vi "terminate.vi"(0 "reference in":refnum<class "Master Controller.lvclass">, 5 "error in (no error)":errorcluster) -> (14 "reference out":refnum<class "Master Controller.lvclass">, 19 "error out":errorcluster)   [LabVIEW 2016, in "Master Controller.lvclass"]
uses:
  Master Controller.lvclass
  File Controller_llb/File Controller.lvclass
  Devices Controller_llb/Devices Controller.lvclass
  Items Controller_llb/Items Controller.lvclass
  PartsTracking Controller_class/PartsTracking Controller.lvclass
  GUI/GUI Controller_llb/GUI Controller.lvclass
  Notification Controller_class/Notification Controller.lvclass
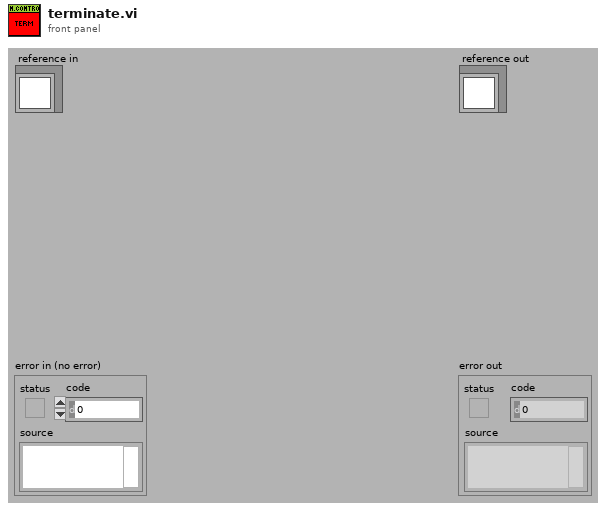
[diagram p1: front panel]
types:
  T1 = typedef "Master Controller.lvclass/ObjectAttributesRef.ctl" = refnum<data-value>
  T2 = typedef "Master Controller.lvclass/ObjectAttributes.ctl" = cluster{"MyAttribute":dbl, "Devices Controller_ref":refnum<class "Devices Controller.lvclass">, "File Controller_ref":refnum<class "File Controller.lvclass">, "Items Controller_ref":refnum<class "Items Controller.lvclass">, "GUI Controller_ref":refnum<class "GUI Controller.lvclass">, "NotificationController_ref":refnum<class "Notification Controller.lvclass">, "PartsTracking Controller_ref":refnum<class "PartsTracking Controller.lvclass">}
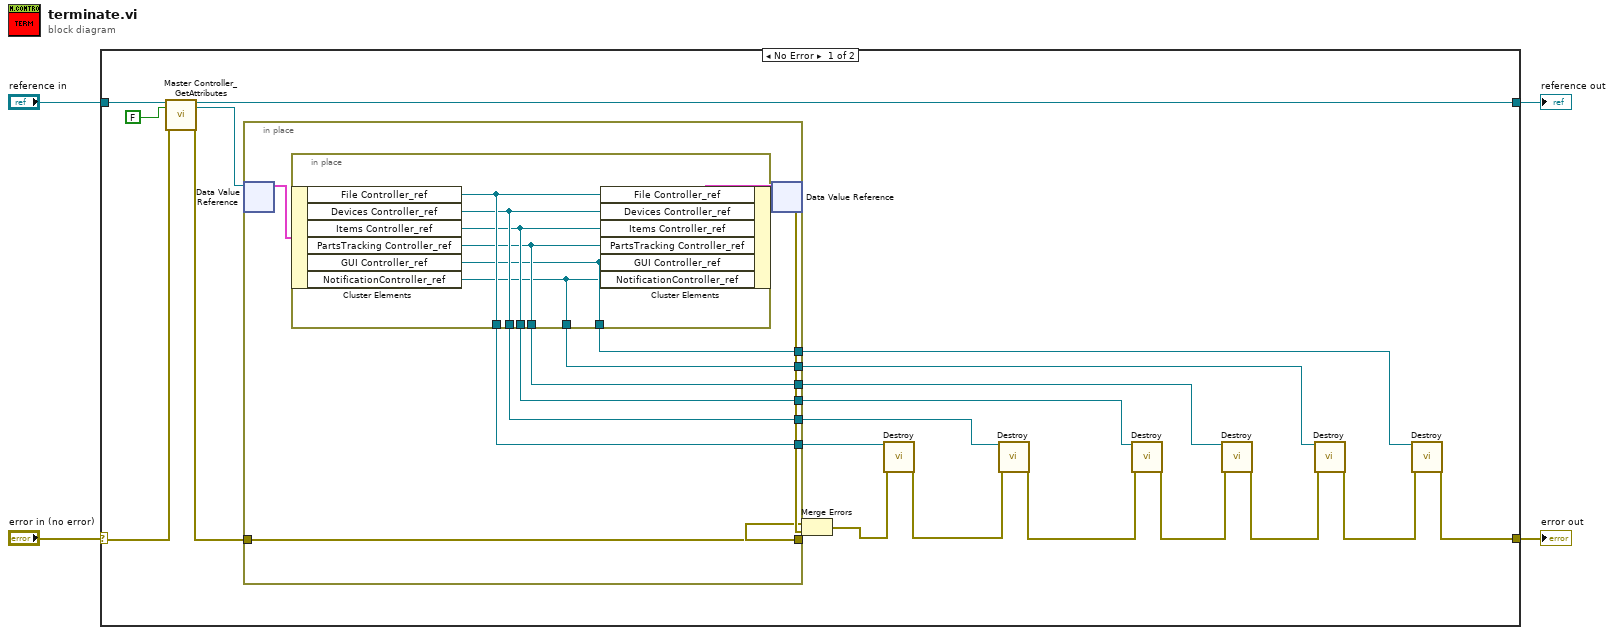
[diagram p0: block diagram]
diagram:
  n1 = case shown="No Error" "error in (no error)" {
    selector: "error in (no error)" -> [w21 w42]
    tunnel: [w8 w42] -> w3
    tunnel: [w19 w41] -> w1
    tunnel: "reference in" -> [w23 w41]
    frame No Error {
      n2 = call "Master Controller_GetAttributes.vi"("reference in"=w23, "return data? (T)"=FALSE, "error in (no error)"=w21) -> ("reference out"=w19:refnum<class "Master Controller.lvclass">, "attributes ref"=w18:T1, "error out"=w20:errorcluster)  [unwired: 13 in, 1 out]
      n3 = in-place {
        in-place-border: w20 -> [w32]
        in-place-border: [w32] -> w24
        in-place-border: [w31] -> w17
        in-place-border: [w30] -> w16
        in-place-border: [w29] -> w13
        in-place-border: [w28] -> w12
        in-place-border: [w27] -> w11
        in-place-border: [w26] -> w7
        n4 = in-place-dvr #1(w18) -> (w33:T2)  [unwired: 1 out]
        n5 = in-place {
          in-place-border: [w40] -> w31
          in-place-border: [w39] -> w30
          in-place-border: [w38] -> w29
          in-place-border: [w37] -> w28
          in-place-border: [w36] -> w27
          in-place-border: [w35] -> w26
          n6 = in-place-cluster #2(w33) -> ("File Controller_ref"=w40:refnum<class "File Controller.lvclass">, "Devices Controller_ref"=w39:refnum<class "Devices Controller.lvclass">, "Items Controller_ref"=w38:refnum<class "Items Controller.lvclass">, "PartsTracking Controller_ref"=w37:refnum<class "PartsTracking Controller.lvclass">, "GUI Controller_ref"=w36:refnum<class "GUI Controller.lvclass">, "NotificationController_ref"=w35:refnum<class "Notification Controller.lvclass">)
          n7 = in-place-cluster #2("File Controller_ref"=w40, "Devices Controller_ref"=w39, "Items Controller_ref"=w38, "PartsTracking Controller_ref"=w37, "GUI Controller_ref"=w36, "NotificationController_ref"=w35) -> (w34:T2)
        }
        n8 = in-place-dvr #1(w34) -> (w25:errorcluster)  [unwired: 1 out]
      }
      n9 = Merge Errors(w24, w25) -> (w14:errorcluster)
      n10 = call-dynamic "Destroy.vi"("reference in"=w17, "error in (no error)"=w14) -> ("error out"=w15:errorcluster)  [unwired: 16 in, 1 out]
      n11 = call-dynamic "Destroy.vi"("reference in"=w16, "error in (no error)"=w15) -> ("error out"=w10:errorcluster)  [unwired: 16 in, 1 out]
      n12 = call-dynamic "Destroy.vi"("reference in"=w13, "error in (no error)"=w10) -> ("error out"=w9:errorcluster)  [unwired: 16 in, 1 out]
      n13 = call-dynamic "Destroy.vi"("reference in"=w12, "error in (no error)"=w9) -> ("error out"=w6:errorcluster)  [unwired: 16 in, 1 out]
      n14 = call-dynamic "Destroy.vi"("reference in"=w7, "error in (no error)"=w6) -> ("error out"=w5:errorcluster)  [unwired: 16 in, 1 out]
      n15 = call-dynamic "Destroy.vi"("reference in"=w11, "error in (no error)"=w5) -> ("error out"=w8:errorcluster)  [unwired: 16 in, 1 out]
    }
    frame Error {
    }
  }
  "error out" <- w3
  "reference out" <- w1
